vi "Init.vi"(8 "error in (no error)":errorcluster) -> (0 "error out":errorcluster, 3 "Controller out":refnum<class "Controller.lvclass">)   [LabVIEW 2020, in "Container.lvlib" / "Controller.lvclass"]
uses:
  Controller.lvclass
  Controller.lvclass/Controller.ctl
  Model/Model/Model.lvclass
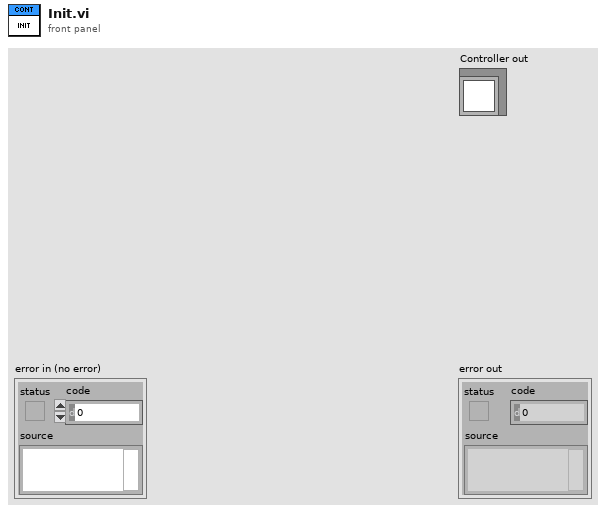
[diagram p1: front panel]
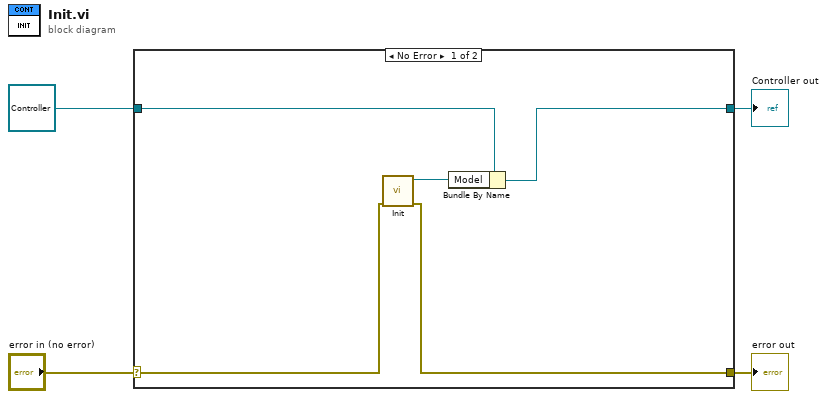
[diagram p0: block diagram]
diagram:
  n1 = case shown="No Error" "error in (no error)" {
    selector: "error in (no error)" -> [w8 w11]
    tunnel: [w9 w11] -> w3
    tunnel: [w6 w10] -> w2
    tunnel: refnum<class "Controller.lvclass"> refnum ("Controller in") -> [w7 w10]
    frame No Error {
      n2 = call "Init.vi"("error in (no error)"=w8) -> ("error out"=w9:errorcluster, "Model out"=w5:refnum<class "Model.lvclass">)  [unwired: 9 in]
      n3 = Bundle By Name(cluster=w7, "Model"=w5) -> (w6:refnum<class "Controller.lvclass">)
    }
    frame Error {
    }
  }
  "error out" <- w3
  "Controller out" <- w2
